vi "WaitForOutput.vi"(8 "error in (no error)":errorcluster, 11 "Subsystem in":refnum<class "Subsystem.lvclass">) -> (0 "error out":errorcluster, 2 "Subsystem Output":refnum<class "SubsystemData.lvclass">, 3 "Subsystem out":refnum<class "Subsystem.lvclass">)   [LabVIEW 2017, in "Subsystem.lvclass"]
uses:
  Subsystem.lvclass
  SubsystemData/SubsystemData.lvclass
  Subsystem.lvclass/Subsystem.ctl
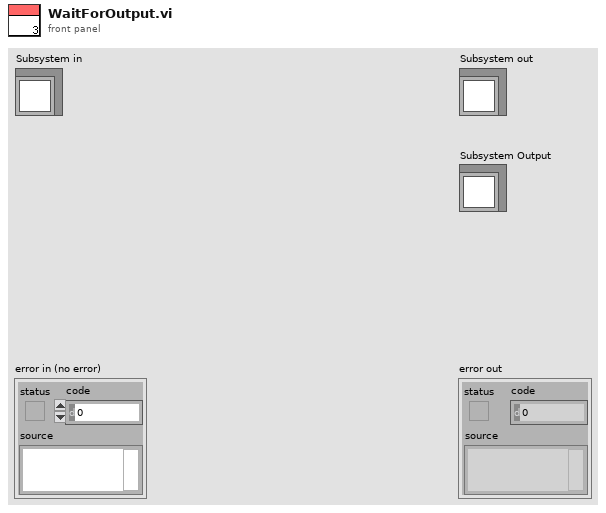
[diagram p1: front panel]
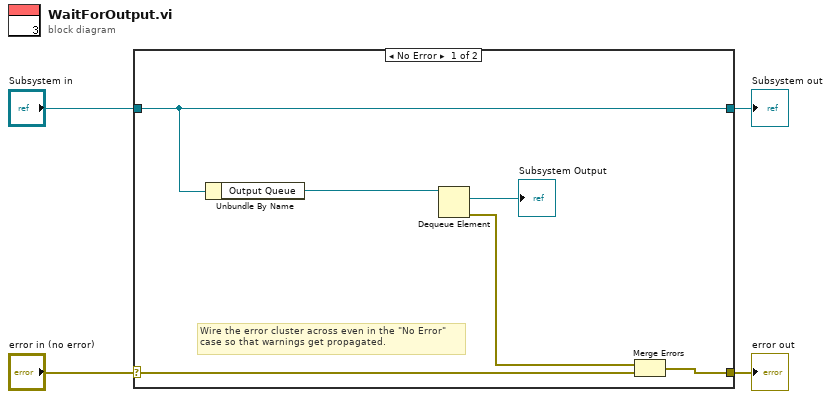
[diagram p0: block diagram]
diagram:
  n1 = case shown="No Error" "error in (no error)" {
    selector: "error in (no error)" -> [w10 w12]
    tunnel: [w7 w12] -> w3
    tunnel: [w8 w11] -> w1
    tunnel: "Subsystem in" -> [w8 w11]
    frame No Error {
      # "Wire the error cluster across even in the \"No Error\"\ncase so that warnings get propagated."
      n2 = Unbundle By Name(w8) -> ("Output Queue"=w9:refnum<queue>)
      n3 = Dequeue Element(queue=w9) -> (element=→"Subsystem Output":refnum<class "SubsystemData.lvclass">, error out=w6:errorcluster)  [unwired: 2 in, 2 out]
      n4 = Merge Errors(w6, w10) -> (w7:errorcluster)
    }
    frame Error {
    }
  }
  "error out" <- w3
  "Subsystem out" <- w1
